vi "time_left_calculator.vi"(10 "Start time":timestamp, 11 "Experiment duration (s)":dbl) -> (0 "Current time":string, 1 "Finish time":timestamp, 2 "Time Left":dbl, 3 "Time has Elapsed":bool)   [LabVIEW 2016]
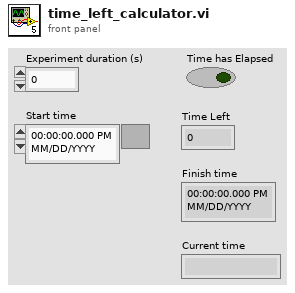
[diagram p1: front panel]
types:
  T1 = typedef "LVDateTimeRec.ctl" = cluster{"fractional second":dbl, "second":i32, "minute":i32, "hour":i32, "day of month":i32, "month":i32, "year":i32, "day of week":i32, "day of year":i32, "DST":i32}
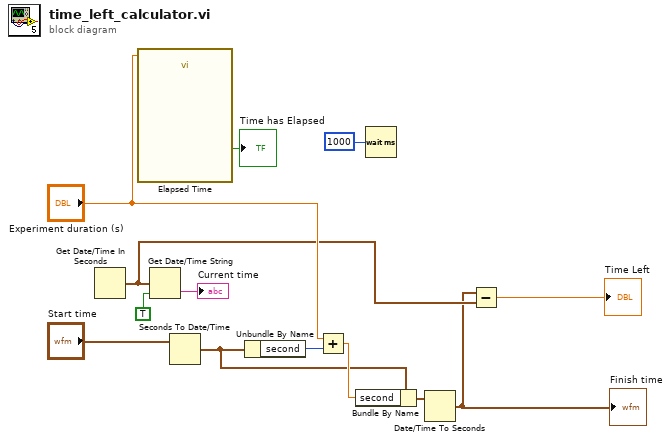
[diagram p0: block diagram]
diagram:
  n1 = Get Date/Time In Seconds() -> (seconds since 1Jan1904=w12:timestamp)
  n2 = call "Elapsed Time"("Time Target (s)"="Experiment duration (s)") -> ("Time has Elapsed"=→"Time has Elapsed":bool)  [unwired: 11 in, 7 out]
  n3 = Get Date/Time String(seconds (now)=w12, want seconds? (F)=TRUE) -> (time string=→"Current time":string)  [unwired: 1 in, 1 out]
  n4 = Seconds To Date/Time(time stamp (now)="Start time") -> (date time rec=w7:T1)  [unwired: 1 in]
  n5 = Unbundle By Name(w7) -> ("second"=w5:i32)
  n6 = Add(x="Experiment duration (s)", y=w5) -> (x+y=w8:dbl)
  n7 = Bundle By Name(cluster=w7, "second"=w8) -> (w9:T1)
  n8 = Wait (ms)(milliseconds to wait=u32 1000) -> ()  [unwired: 1 out]
  n9 = Date/Time To Seconds(2:w9) -> (0:w11:timestamp)  [unwired: 1 in]
  "Finish time" <- w11
  n10 = Subtract(x=w11, y=w12) -> (x-y=→"Time Left":dbl)
